vi "ConvertStringToTimestamp.vi"(1 "DateTimeString":string) -> (0 "TimeStamp":timestamp)   [LabVIEW 2018]
doc: "This VI convert a date/time string back to a time stamp.\n\nCopyright © 2011 Epimedia, Inc. All Rights Reserved.\n\nThe Epimedia Application Library is Copyright © 2009-2011 Epimedia, Inc. \nAll Rights Reserved. Used under license."
panel:
  # "This control should have data in the form:\n4/30/2004 7:48:47\nCaveat:  use 24 hour time format, such that 12:00 AM is 00:00."
  # "Copyright © 2011 Epimedia, Inc. All Rights Reserved.\n\nThe Epimedia Application Library is Copyright © 2009-2011 Epimedia, Inc. \nAll Rights Reserved. Used under license."
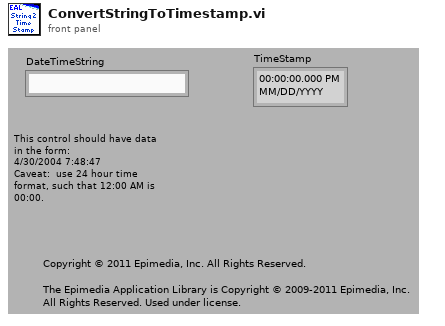
[diagram p1: front panel]
types:
  T1 = cluster{"second":i32, "minute":i32, "hour":i32, "day of month":i32, "month":i32, "year":i32, "day of week":i32, "day of year":i32, "is DST":i32}
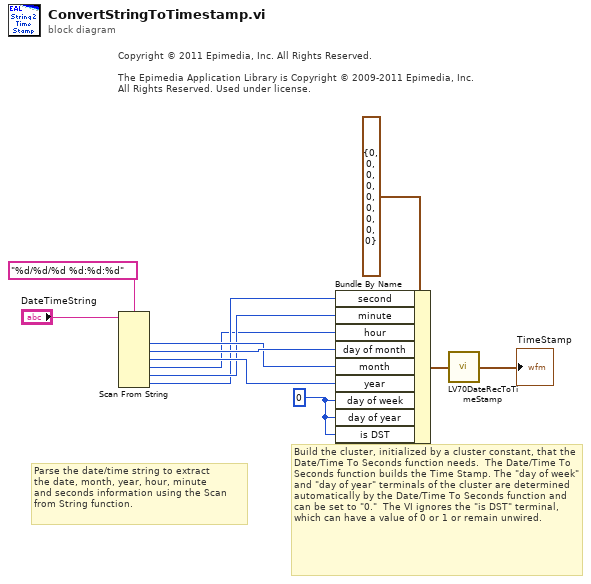
[diagram p0: block diagram]
diagram:
  w7 = 0
  # "Copyright © 2011 Epimedia, Inc. All Rights Reserved.\n\nThe Epimedia Application Library is Copyright © 2009-2011 Epimedia, Inc. \nAll Rights Reserved. Used under license."
  # "Build the cluster, initialized by a cluster constant, that the Date/Time To Seconds function needs.  The Date/Time To Seconds function builds the Time Stamp. The \"day of week\" and \"day of year\" terminals of the cluster are determined automatically by the Date/Time To Seconds function and can be set to \"0.\"  The VI ignores the \"is DST\" terminal, which can have a value of 0 or 1 or remain unwired."
  # "Parse the date/time string to extract \nthe date, month, year, hour, minute \nand seconds information using the Scan\nfrom String function."
  n1 = Scan From String "Scan From String"(format string="%d/%d/%d %d:%d:%d", input string="DateTimeString") -> (output 1=w5:i32, output 2=w6:i32, output 3=w4:i32, output 4=w1:i32, output 5=w3:i32, output 6=w2:i32)  [unwired: 2 in, 9 out]
  n2 = Bundle By Name(cluster=T1 {"second"=0, "minute"=0, "hour"=0, "day of month"=0, "month"=0, "year"=0, "day of week"=0, "day of year"=0, "is DST"=0} ("date time rec"), "second"=w2, "minute"=w3, "hour"=w1, "day of month"=w6, "month"=w5, "year"=w4, "day of week"=w7, "day of year"=w7, "is DST"=w7) -> (w8:T1)
  n3 = call <vilib>:"LV70DateRecToTimeStamp.vi"("date time rec"=w8) -> ("Time Stamp"=→"TimeStamp":timestamp)
